vi "PC_Pub_imgFile updFilePath.vi"(8 "error in (no error)":errorcluster, 11 "imgFile in":refnum<class "PC_Pub_imgFile.lvclass">) -> (0 "error out":errorcluster, 3 "imgFile out":refnum<class "PC_Pub_imgFile.lvclass">)   [LabVIEW 2018, in "PC_Pub_imgFile.lvclass"]
uses:
  PC_Pub_imgFile.lvclass
  PC_Pub_imgFile.lvclass/PC_Pub_imgFile.ctl
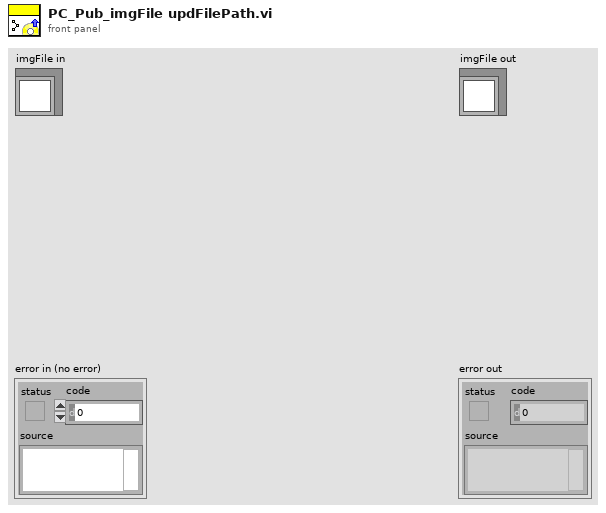
[diagram p1: front panel]
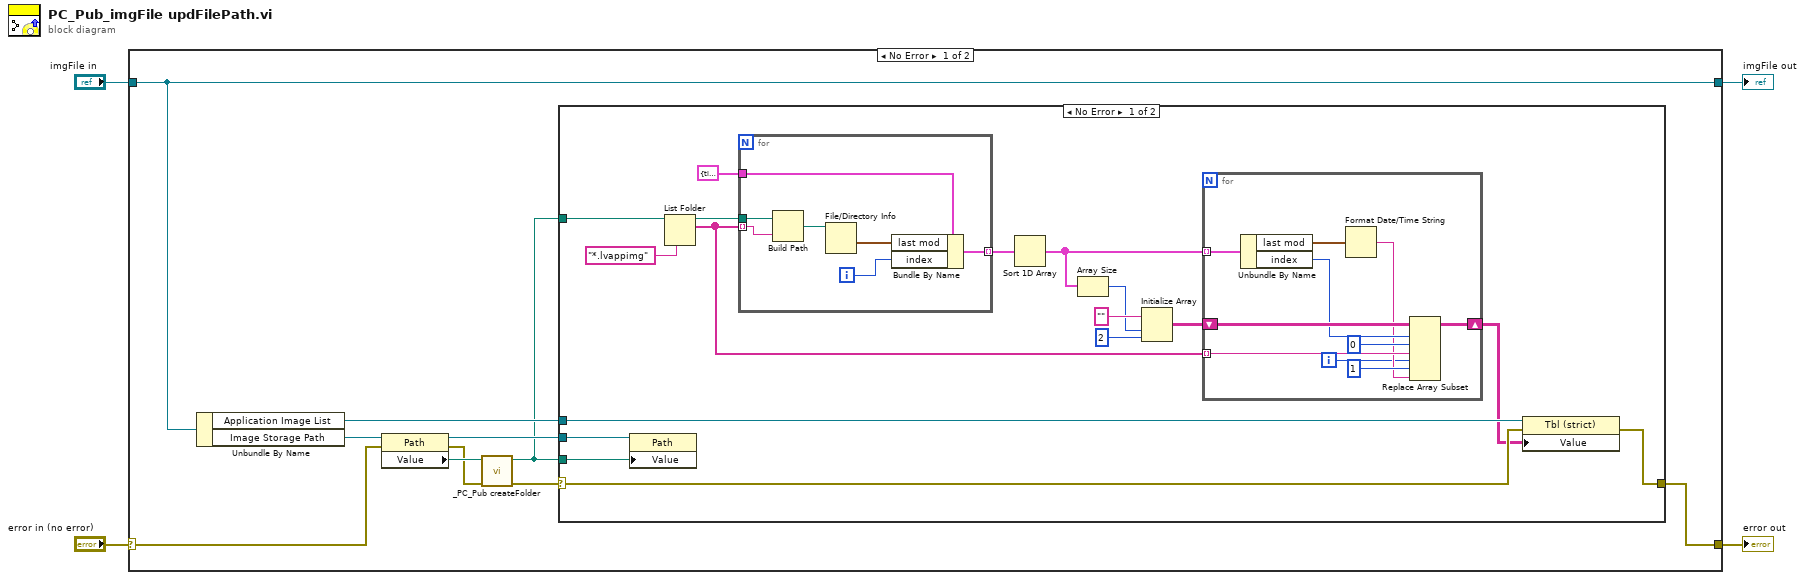
[diagram p0: block diagram]
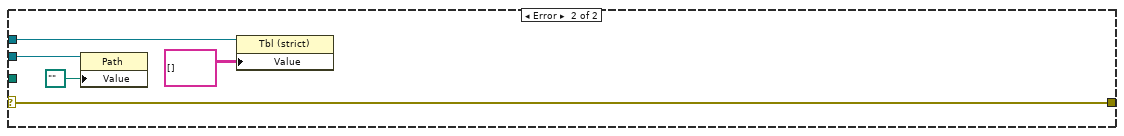
[diagram p2: hidden frame]
diagram:
  n1 = case shown="No Error" "error in (no error)" {
    selector: "error in (no error)" -> [w12 w55]
    tunnel: [w8 w55] -> w3
    tunnel: [w7 w54] -> w1
    tunnel: "imgFile in" -> [w7 w54]
    frame No Error {
      n2 = Unbundle By Name(w7) -> ("Application Image List"=w9:refnum<vi>, "Image Storage Path"=w14:refnum<vi>)
      n3 = property class="Path"(reference=w14, error in=w12) -> (reference out=w6:refnum<vi>, error out=w11:errorcluster, "Value"=w13:path)
      n4 = call "_PC_Pub createFolder.vi"("error in (no error)"=w11, "path (use dialog)"=w13) -> ("error out"=w10:errorcluster, "created path"=w5:path)  [unwired: 8 in]
      n5 = case shown="No Error" w10 {
        selector: w10 -> [w30 w53]
        tunnel: w9 -> [w31 w50]
        tunnel: w5 -> [w15 _]
        tunnel: [w29 w53] -> w8
        tunnel: w6 -> [w28 w52]
        tunnel: w5 -> [w27 _]
        frame No Error {
          n6 = property class="Path"(reference=w28, "Value"=w27) -> ()  [unwired: 1 in, 2 out]
          n7 = List Folder(path=w15, pattern="*.lvappimg") -> (path out=w25:path, filenames=w17:string[])  [unwired: 2 in, 2 out]
          n8 = for {
            tunnel: w25 -> [w47]
            tunnel: w17 -> [w46] mode=indexing
            tunnel: cluster{"last mod":timestamp, "index":i32} {"last mod"=timestamp(0 s since 1904-01-01), "index"=0} -> [w45]
            tunnel: [w43] -> w23 mode=indexing
            i -> [w42]
            n9 = Build Path(base path=w47, name or relative path=w46) -> (appended path=w48:path)
            n10 = File/Directory Info(path=w48) -> (last mod=w44:timestamp)  [unwired: 1 in, 6 out]
            n11 = Bundle By Name(cluster=w45, "last mod"=w44, "index"=w42) -> (w43:cluster{"last mod":timestamp, "index":i32})
          }
          n12 = Sort 1D Array(array=w23) -> (sorted array=w20:cluster{"last mod":timestamp, "index":i32}[])
          n13 = Array Size(array=w20) -> (size(s)=w21:i32)
          n14 = Initialize Array("", w21, 2 ("dimension size")) -> (w19:string[][])
          n15 = for {
            tunnel: w20 -> [w40] mode=indexing
            shift-right: [w39] -> w16
            shift-left: w19 -> [w41]
            tunnel: w17 -> [w34] mode=indexing
            i -> [w32]
            n16 = Unbundle By Name(w40) -> ("last mod"=w38:timestamp, "index"=w37:i32)
            n17 = Format Date/Time String(seconds (now)=w38) -> (date/time string=w33:string)  [unwired: 2 in]
            n18 = Replace Array Subset(array=w41, new element #1=w34, index (row) #1=w37, index (col) #1=0 ("disabled index (col)"), new element #2=w33, index (row) #2=w32, index (col) #2=1 ("disabled index (col)")) -> (w39:string[][])
          }
          n19 = property class="Tbl (strict)"(reference=w31, error in=w30, "Value"=w16) -> (error out=w29:errorcluster)  [unwired: 1 out]
        }
        frame Error {
          n20 = property class="Path"(reference=w52, "Value"=path "") -> ()  [unwired: 1 in, 2 out]
          n21 = property class="Tbl (strict)"(reference=w50, "Value"=string[][] []) -> ()  [unwired: 1 in, 2 out]
        }
      }
    }
    frame Error {
    }
  }
  "error out" <- w3
  "imgFile out" <- w1
